vi "New Face.vi"(8 "error in (no error)":errorcluster, 9 "index (first)":i32, 10 "Path":path, 11 "library in":i64) -> (0 "error out":errorcluster, 2 "face out":i64, 3 "library out":i64)   [LabVIEW 2023, in "Freetype Drawer.lvlib"]
uses:
  Freetype Drawer.lvlib
  libfreetype.dll
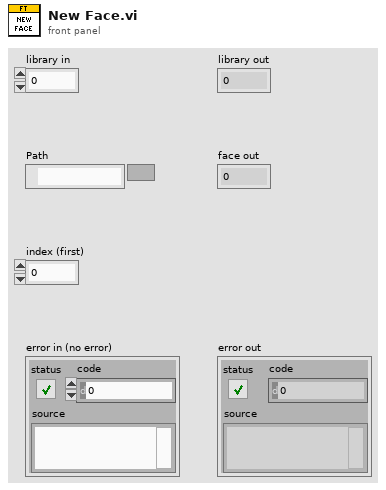
[diagram p1: front panel]
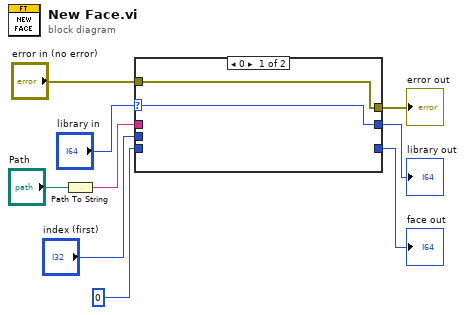
[diagram p0: block diagram]
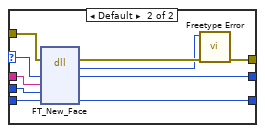
[diagram p2: hidden frame]
diagram:
  n1 = Path To String(path="Path") -> (string=w2:string)
  n2 = case shown="0" "library in" {
    selector: "library in" -> [w10 w17]
    tunnel: "error in (no error)" -> [w11 w21]
    tunnel: i64 0 ("face") -> [_ w20]
    tunnel: "index (first)" -> [_ w19]
    tunnel: [_ w18] -> w5
    tunnel: [w10 w16] -> w3
    tunnel: w2 -> [_ w15]
    tunnel: [w11 w12] -> w1
    frame 0 {
    }
    frame Default {
      n3 = dll-call lib="E:/Labview/LV 2023/Libs/LV Symbol/Freetype Drawer/libfreetype.dll" fn="FT_New_Face"(error in=w21, "library"=w17, "path"=w15, "index"=w19, "face"=w20) -> (error out=w14:errorcluster, "error"=w13:i32, "library"=w16:i64, "face"=w18:i64)  [unwired: 4 in, 1 out]
      n4 = call "Freetype Error.vi"("error in (no error)"=w14, "Error"=w13) -> ("error out"=w12:errorcluster)  [unwired: 9 in]
    }
  }
  "face out" <- w5
  "error out" <- w1
  "library out" <- w3
